vi "ISEG_HVSystem.ProcCases.vi"(0 "i ref in":refnum<vi>, 1 "selector":string, 2 "Data":T1, 3 "call cluster":T2={"Object"="", "Selector"="", "CallType"=enum."synchronous", "Async Object"="", "Async Selector"="", "Data Descriptor"="", "Data"=[], "Error #"=0, "Expire"=0}, 5 "error in (no error)":errorcluster) -> (14 "i ref out":refnum<vi>, 17 "answer cluster":T2={"Object"="", "Selector"="", "CallType"=enum."synchronous", "Async Object"="", "Async Selector"="", "Data Descriptor"="", "Data"=[], "Error #"=0, "Expire"=0}, 19 "error out":errorcluster)   [LabVIEW 2014, in "ISEG_HVSystem.lvlib"]
doc: "This method is called by a process from within the default case in the event loop. The methods of a class that are linked to events will be called from THIS method. Add your code here."
uses:
  ISEG_HVSystem.lvlib
  CSCore/CSSystem/CoreDefs/CoreDefs.call_type.ctl
  CSCore/BaseProcess/BaseProcess.descriptor string definition.ctl
  CSCore/CSSystem/CoreDefs/CoreDefs.rawDataType.ctl
  CSCore/CSSystem/CoreLib/CoreLib.byte array 2 string.vi
  CSCore/CSSystem/CoreLib/CoreLib.string 2 byte array.vi
  CSCore/CSSystem/CoreLib/CoreLib.byte array 2 short.vi
  CSCore/CSSystem/CoreLib/CoreLib.short 2 byte array.vi
  CSCore/CSSystem/CoreLib/CoreLib.byte array 2 double.vi
  CSCore/CSSystem/CoreLib/CoreLib.double 2 byte array.vi
  CSCore/CSApplicationBaseClasses/DeviceBase/DeviceBase.lvlib
  CSCore/CSSystem/CoreLib/CoreLib.lvlib
  CSCore/BaseProcess/BaseProcess.lvlib
  CSCore/CAEObj/CAEObj.lvlib
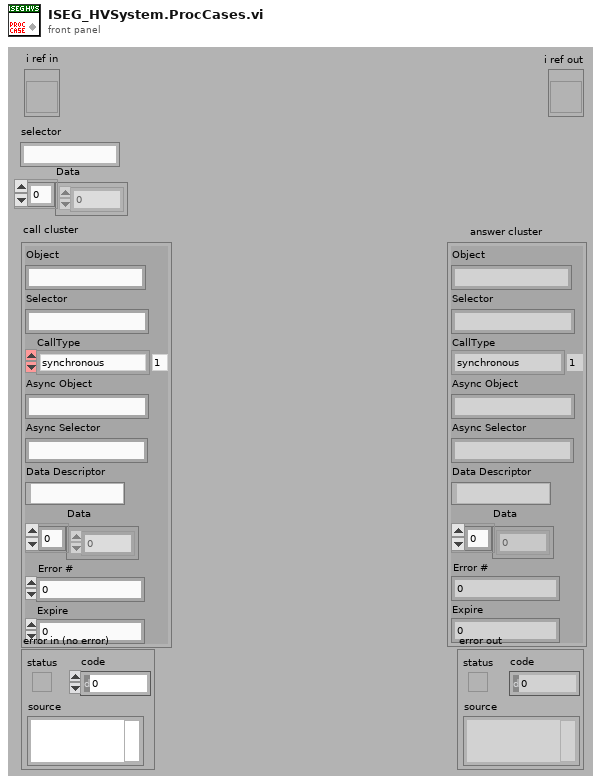
[diagram p1: front panel]
types:
  T1 = typedef "CoreDefs.rawDataType.ctl" = i8[]
  T2 = typedef "CoreDefs.call_type.ctl" = cluster{"Object":string, "Selector":string, "CallType":enum16{"simple", "synchronous", "asynchronous"}, "Async Object":string, "Async Selector":string, "Data Descriptor":T3, "Data":T1, "Error #":i32, "Expire":u32}
  T3 = typedef "BaseProcess.lvlib/BaseProcess.descriptor string definition.ctl" = string
  T4 = typedef "BaseProcess.lvlib/BaseProcess.i attribute.ctl" = cluster{"EventStatus":string, "EventError":i32, "PresetEvtWatchD":i32, "PresetPdcWatchD":i32, "EventTimeout":i32, "PeriodicInterval":i32, "Interface":string[], "Address":string[], "Special":string[], "PeriodicError":i32, "PeriodicStatus":string, "SuperProc":string, "Descriptors":T5[], "CaseRef":refnum<vi>, "PdcRef":refnum<vi>, "Thread Ref":refnum<vi>, "eventErrorID":i32, "eventStatusID":i32, "periodicErrorID":i32, "periodicStatusID":i32, "pdcCtrID":i32}
  T5 = typedef "BaseProcess.lvlib/BaseProcess.descriptor definition.ctl" = cluster{"selector":string, "descriptor":T3}
  T6 = typedef "ISEG_HVSystem.lvlib/ISEG_HVSystem.i attribute.ctl" = cluster{"System Name":string, "CAN_Status bus":cluster{"CAN":string, "DIM Status":T7}, "Client Active?":cluster{"Active":bool, "DIM Status":T7}, "Client Connected?":cluster{"Connected":bool, "DIM Status":T7}, "OPC Version":cluster{"OPC Version":string, "DIM Status":T7}, "Pr ID":cluster{"Pr ID":string, "DIM Status":T7}, " Modell":string, " Prefix":string, "Force":cluster{"Force":bool, "DIM Status":T7}, "Refresh":cluster{"Refresh":dbl, "DIM Status":T7}}
  T7 = typedef "ISEG_HVSystem.lvlib/ISEG_HVSystem.DIM Status.ctl" = cluster{"no link":bool, "quality":i32, "Time Stamp":timestamp}
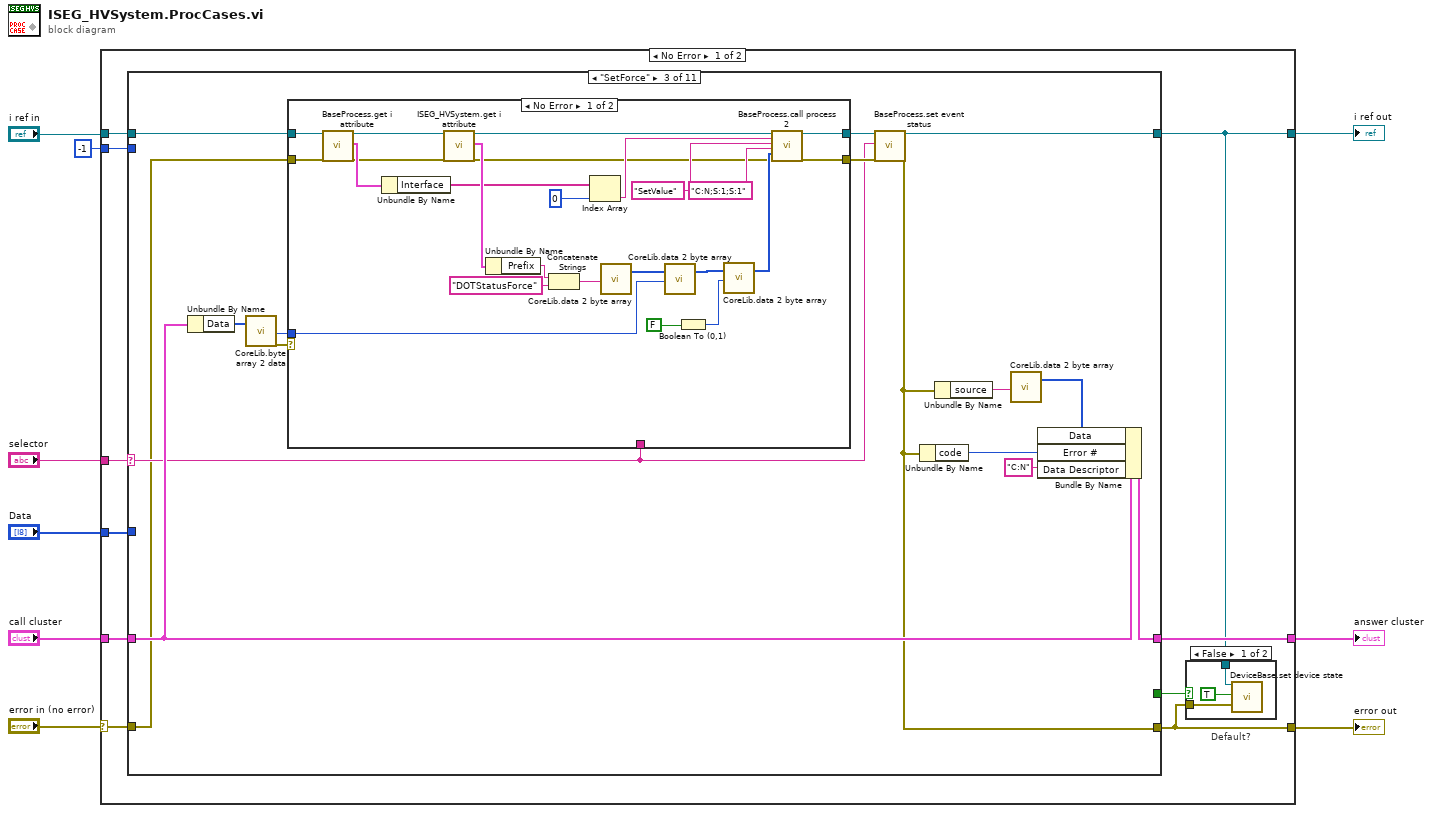
[diagram p0: block diagram]
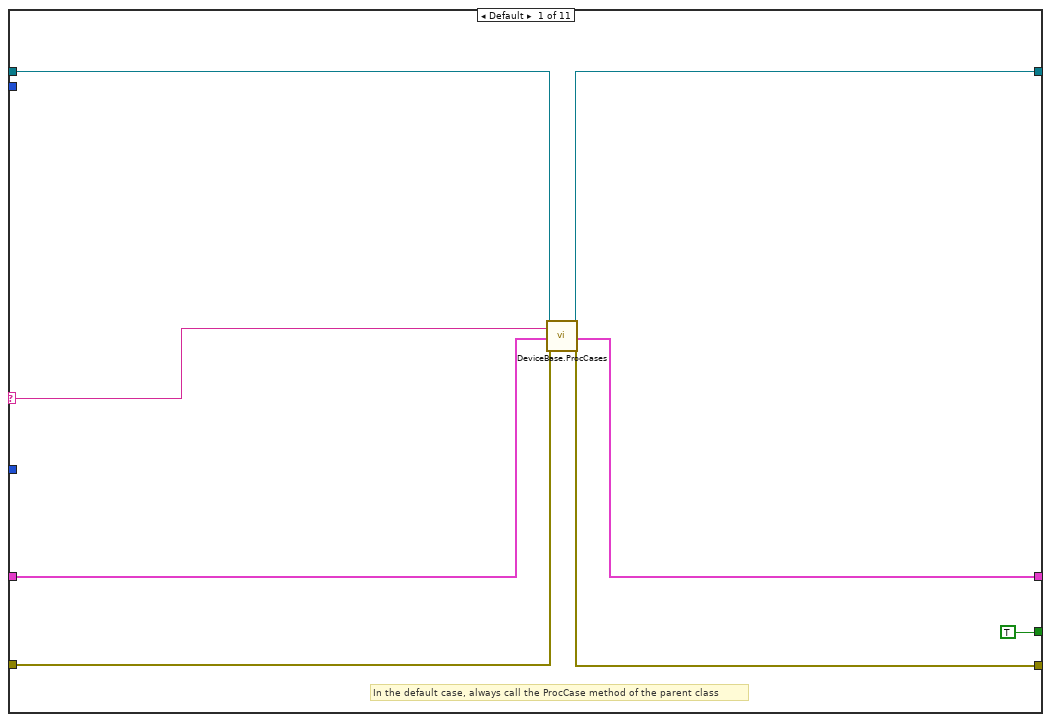
[diagram p3: hidden frame]
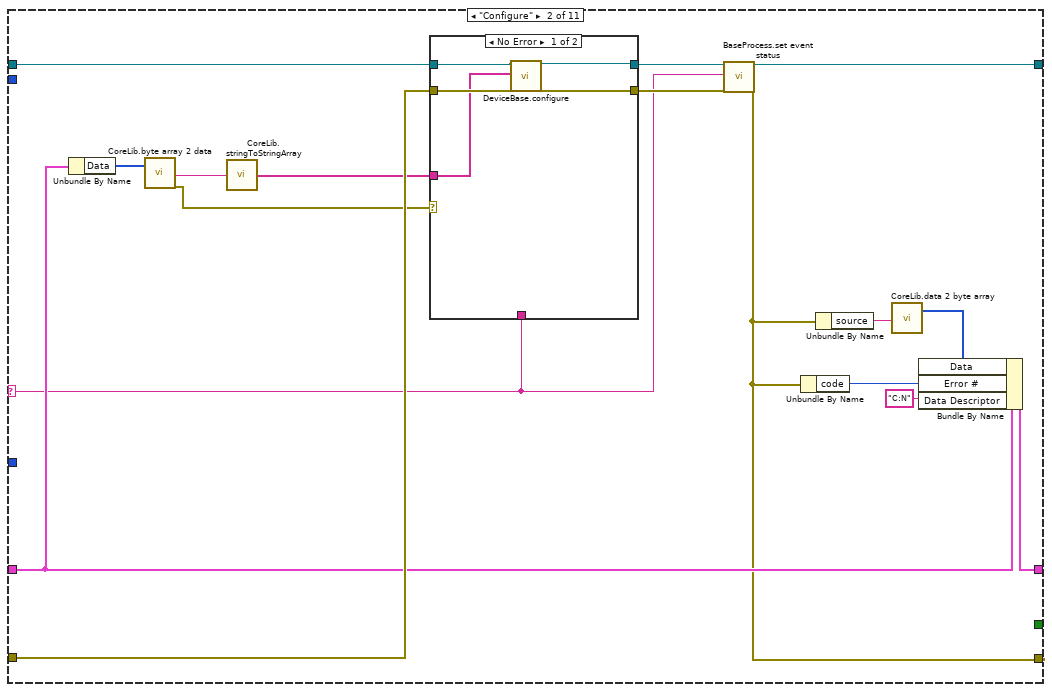
[diagram p4: hidden frame]
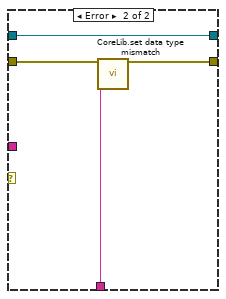
[diagram p5: hidden frame]
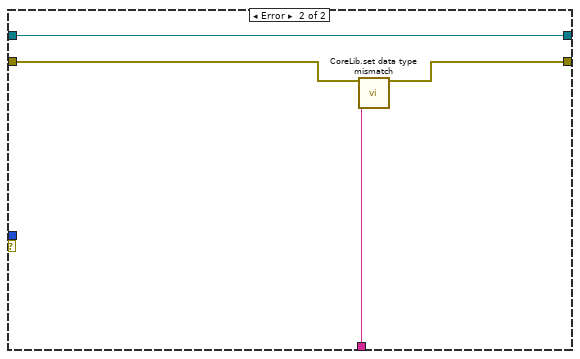
[diagram p6: hidden frame]
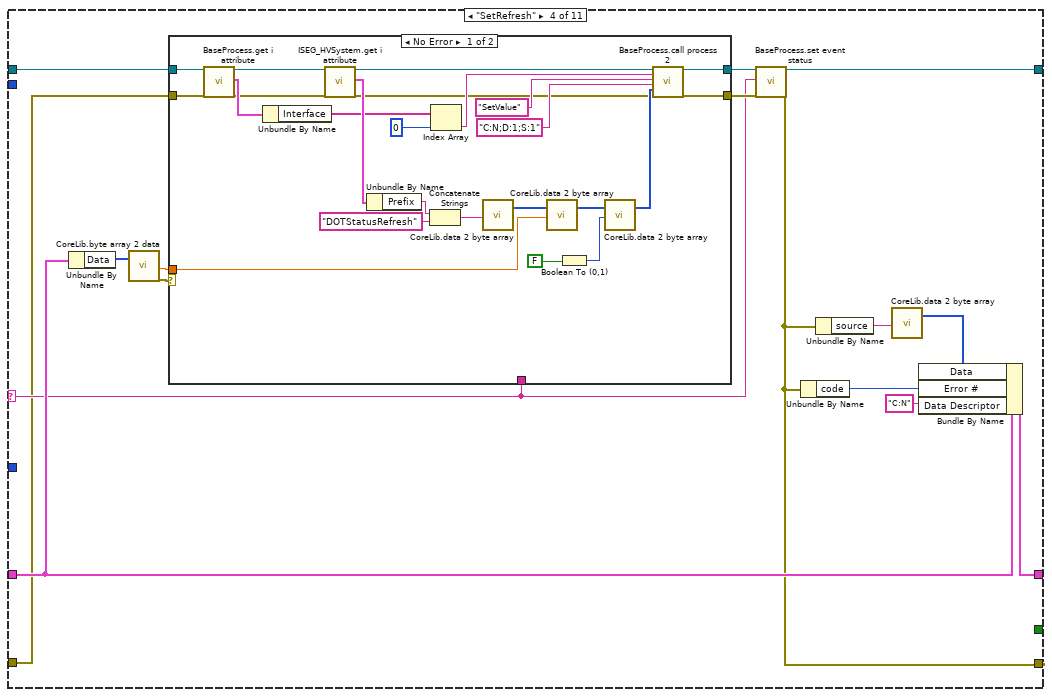
[diagram p7: hidden frame]
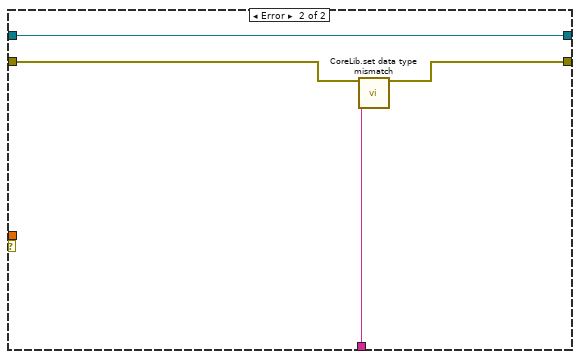
[diagram p8: hidden frame]
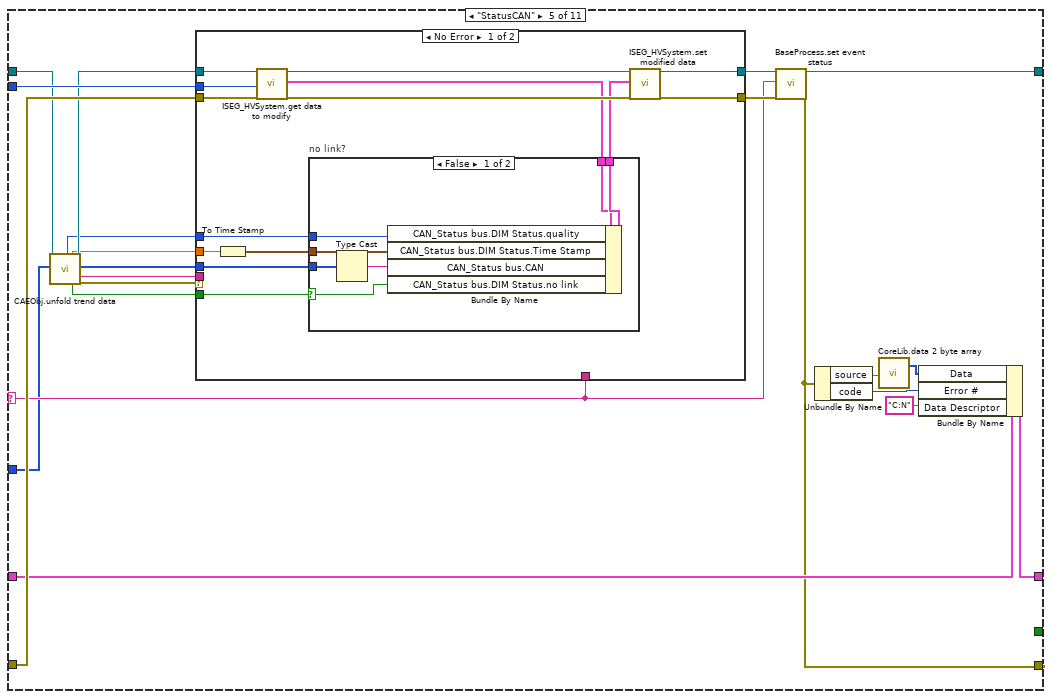
[diagram p9: hidden frame]
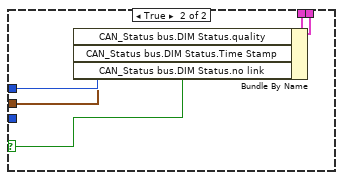
[diagram p10: hidden frame]
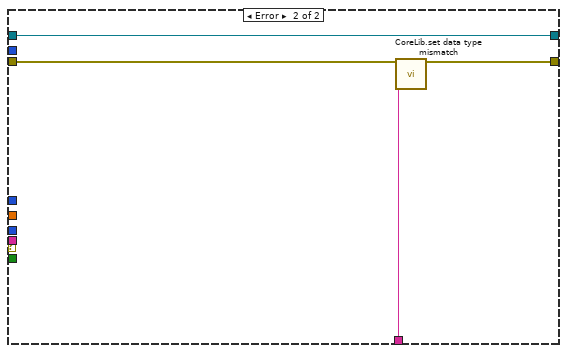
[diagram p11: hidden frame]
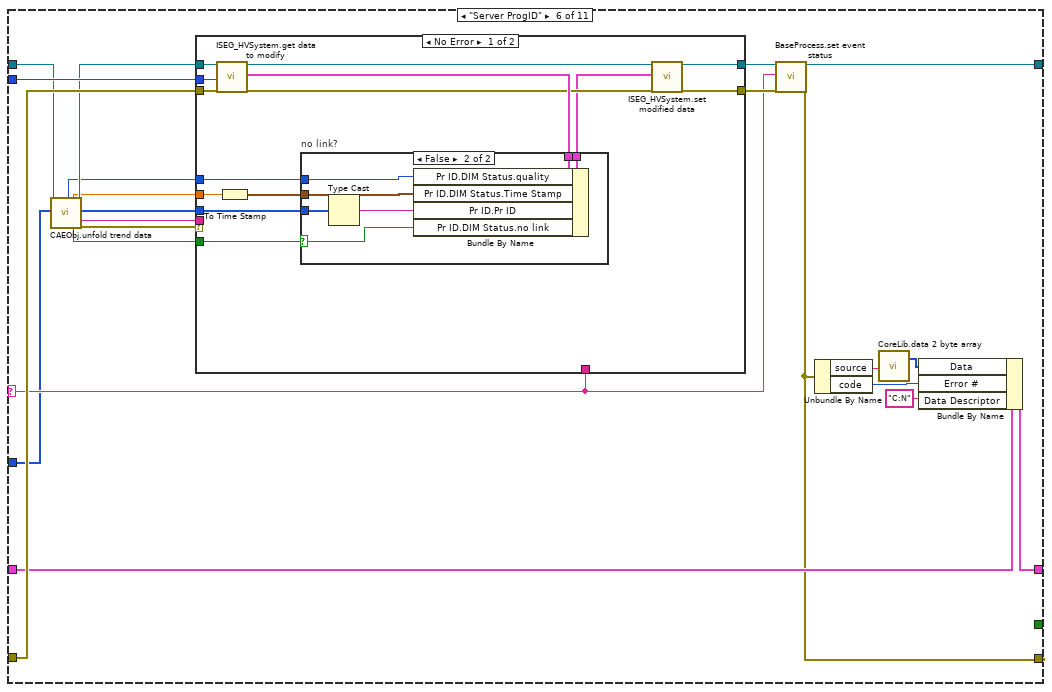
[diagram p12: hidden frame]
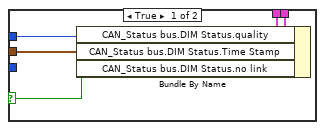
[diagram p13: hidden frame]
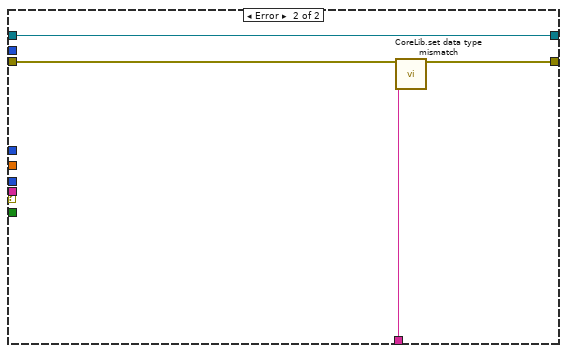
[diagram p14: hidden frame]
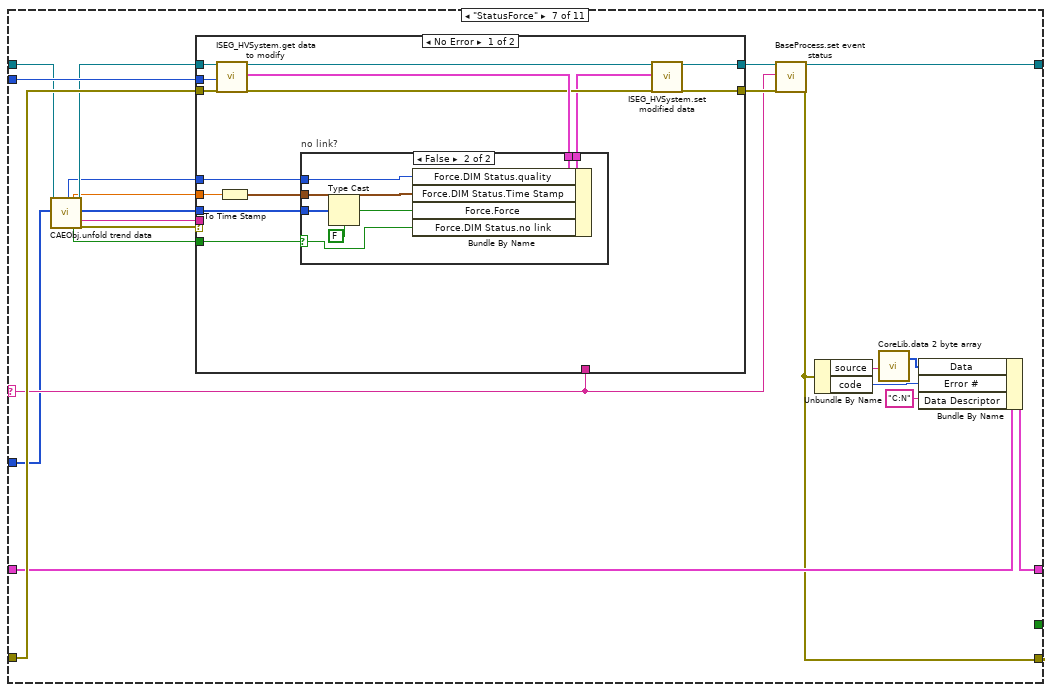
[diagram p15: hidden frame]
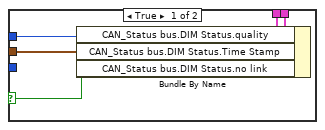
[diagram p16: hidden frame]
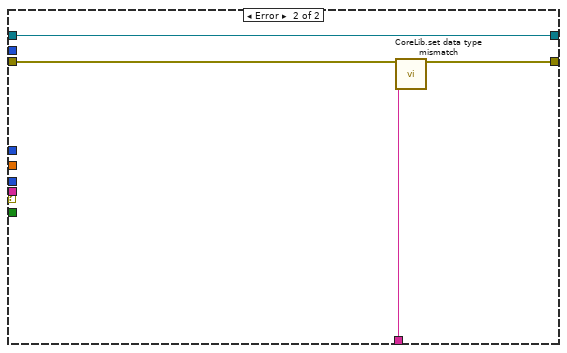
[diagram p17: hidden frame]
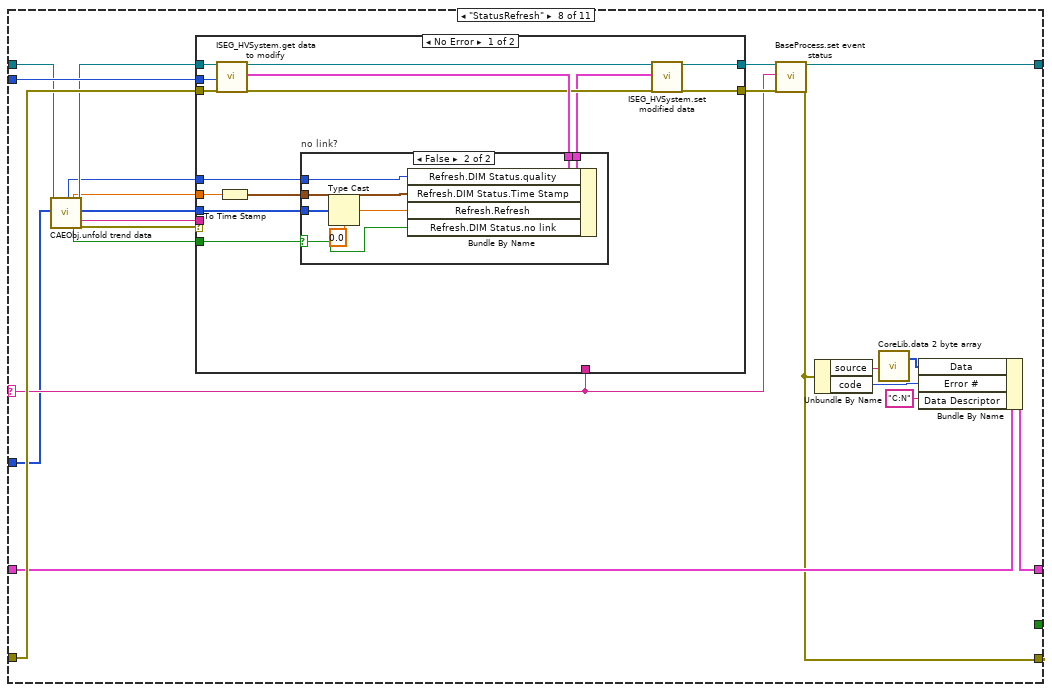
[diagram p18: hidden frame]
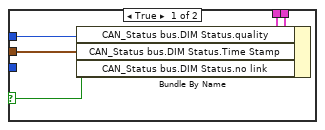
[diagram p19: hidden frame]
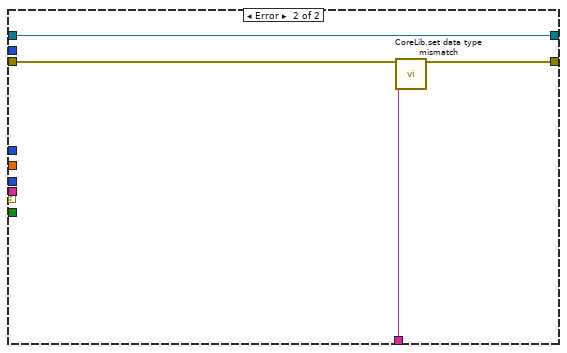
[diagram p20: hidden frame]
diagram:
  n1 = case shown="No Error" "error in (no error)" {
    selector: "error in (no error)" -> [w14 w512]
    tunnel: "selector" -> [w19 _]
    tunnel: [w18 w513] -> w3
    tunnel: "Data" -> [w17 _]
    tunnel: "call cluster" -> [w16 w513]
    tunnel: "i ref in" -> [w15 w514]
    tunnel: [w10 w514] -> w1
    tunnel: [w12 w512] -> w2
    tunnel: -1 ("ms timeout (10000)") -> [w13 _]
    frame No Error {
      n2 = case shown="\"SetForce\"" w19 {
        selector: w19 -> [w25 w38 w63 w107 w157 w209 w261 w314 w367 w419 w472]
        tunnel: w17 -> [_ _ _ _ w153 w205 w257 w310 w363 w415 w468]
        tunnel: w15 -> [w24 w47 w71 w115 w152 w204 w256 w309 w362 w414 w467]
        tunnel: [w30 w37 w62 w106 w156 w208 w260 w313 w366 w418 w471] -> w10
        tunnel: w16 -> [w26 w44 w69 w113 w163 w215 w267 w320 w373 w425 w478]
        tunnel: [w27 w43 w68 w112 w162 w214 w266 w319 w372 w424 w477] -> w18
        tunnel: w14 -> [w29 w46 w59 w103 w165 w217 w269 w322 w375 w427 w480]
        tunnel: [w28 w39 w64 w108 w158 w210 w262 w315 w368 w420 w473] -> w12
        tunnel: w13 -> [_ _ _ _ w154 w206 w258 w311 w364 w416 w469]
        tunnel: [TRUE _ _ _ _ _ _ _ _ _ _] -> w11
        frame Default {
          # "In the default case, always call the ProcCase method of the parent class"
          n3 = call "DeviceBase.ProcCases.vi"("i ref in"=w24, "selector"=w25, "call cluster"=w26, "error in (no error)"=w29) -> ("i ref out"=w30:refnum<vi>, "answer cluster"=w27:T2, "error out"=w28:errorcluster)  [unwired: 13 in]
        }
        frame "Configure" {
          n4 = Unbundle By Name(w44) -> ("Data"=w35:T1)
          n5 = call-poly "CoreLib.byte array 2 data.vi"("byteArray"=w35) -> ("string"=w32:string, "error out"=w33:errorcluster)  [unwired: 16 in, 1 out]
          n6 = call "CoreLib.stringToStringArray.vi"("String"=w32) -> ("Array"=w31:string[])
          n7 = case shown="No Error" w33 {
            tunnel: [w49 w55] -> w41
            tunnel: w47 -> [w50 w55]
            tunnel: w46 -> [w51 w54]
            tunnel: [w51 w53] -> w40
            tunnel: w38 -> [_ w52]
            tunnel: w31 -> [w48 _]
            frame No Error {
              n8 = call "DeviceBase.configure.vi"("i ref in"=w50, "configureData"=w48) -> ("i ref out"=w49:refnum<vi>)  [unwired: 15 in, 2 out]
            }
            frame Error {
              n9 = call "CoreLib.set data type mismatch.vi"("error in (no error)"=w54, "error source"=w52) -> ("error out"=w53:errorcluster)  [unwired: 17 in]
            }
          }
          n10 = call "BaseProcess.set event status.vi"("i ref in"=w41, "EventStatus"=w38, "error in (no error)"=w40) -> ("i ref out"=w37:refnum<vi>, "error out"=w39:errorcluster)  [unwired: 14 in, 1 out]
          n11 = Unbundle By Name(w39) -> ("code"=w45:i32)
          n12 = Unbundle By Name(w39) -> ("source"=w34:string)
          n13 = call-poly "CoreLib.data 2 byte array.vi"("string"=w34) -> ("byteArray out"=w42:T1)  [unwired: 18 in]
          n14 = Bundle By Name(cluster=w44, "Data"=w42, "Error #"=w45, "Data Descriptor"="C:N") -> (w43:T2)
        }
        frame "SetForce" {
          n15 = Unbundle By Name(w69) -> ("Data"=w58:T1)
          n16 = call-poly "CoreLib.byte array 2 data.vi"("byteArray"=w58) -> ("i16"=w57:i16, "error out"=w56:errorcluster)  [unwired: 16 in, 1 out]
          n17 = case shown="No Error" w56 {
            tunnel: [w78 w99] -> w66
            tunnel: w71 -> [w95 w99]
            tunnel: w59 -> [w94 w98]
            tunnel: [w79 w97] -> w65
            tunnel: w63 -> [_ w96]
            tunnel: w57 -> [w73 _]
            frame No Error {
              n18 = call "BaseProcess.get i attribute.vi"("i ref in"=w95, "error in (no error)"=w94) -> ("i ref out"=w92:refnum<vi>, "i attribute"=w93:T4, "error out"=w91:errorcluster)  [unwired: 15 in]
              n19 = Unbundle By Name(w93) -> ("Interface"=w84:string[])
              n20 = call "ISEG_HVSystem.get i attribute.vi"("i ref in"=w92, "error in (no error)"=w91) -> ("i ref out"=w77:refnum<vi>, "i attribute"=w90:T6, "error out"=w80:errorcluster)  [unwired: 15 in]
              n21 = Unbundle By Name(w90) -> ("Prefix"=w89:string)
              n22 = Concatenate Strings(w89, "DOTStatusForce" ("string")) -> (w87:string)
              n23 = Index Array(array=w84, index=0) -> (element=w85:string)
              n24 = call-poly "CoreLib.data 2 byte array.vi"("string"=w87) -> ("byteArray out"=w74:T1)  [unwired: 18 in]
              n25 = call-poly "CoreLib.data 2 byte array.vi"("byteArray"=w74, "i16"=w73) -> ("byteArray out"=w72:T1)  [unwired: 17 in]
              n26 = Boolean To (0,1)(Boolean=FALSE) -> (0, 1=w75:i16)
              n27 = call-poly "CoreLib.data 2 byte array.vi"("byteArray"=w72, "i16"=w75) -> ("byteArray out"=w81:T1)  [unwired: 17 in]
              n28 = call "BaseProcess.call process 2.vi"("i ref in"=w77, "Object"=w85, "Selector"="SetValue", "Data Descriptor"="C:N;S:1;S:1", "Data"=w81, "error in (no error)"=w80) -> ("i ref out"=w78:refnum<vi>, "error out"=w79:errorcluster)  [unwired: 12 in]
            }
            frame Error {
              n29 = call "CoreLib.set data type mismatch.vi"("error in (no error)"=w98, "error source"=w96) -> ("error out"=w97:errorcluster)  [unwired: 17 in]
            }
          }
          n30 = call "BaseProcess.set event status.vi"("i ref in"=w66, "EventStatus"=w63, "error in (no error)"=w65) -> ("i ref out"=w62:refnum<vi>, "error out"=w64:errorcluster)  [unwired: 14 in, 1 out]
          n31 = Unbundle By Name(w64) -> ("code"=w70:i32)
          n32 = Unbundle By Name(w64) -> ("source"=w60:string)
          n33 = call-poly "CoreLib.data 2 byte array.vi"("string"=w60) -> ("byteArray out"=w67:T1)  [unwired: 18 in]
          n34 = Bundle By Name(cluster=w69, "Data"=w67, "Error #"=w70, "Data Descriptor"="C:N") -> (w68:T2)
        }
        frame "SetRefresh" {
          n35 = Unbundle By Name(w113) -> ("Data"=w100:T1)
          n36 = call-poly "CoreLib.byte array 2 data.vi"("byteArray"=w100) -> ("d64"=w102:dbl, "error out"=w101:errorcluster)  [unwired: 16 in, 1 out]
          n37 = case shown="No Error" w101 {
            tunnel: [w122 w143] -> w110
            tunnel: w115 -> [w139 w143]
            tunnel: w103 -> [w138 w142]
            tunnel: [w123 w141] -> w109
            tunnel: w107 -> [_ w140]
            tunnel: w102 -> [w116 _]
            frame No Error {
              n38 = call "BaseProcess.get i attribute.vi"("i ref in"=w139, "error in (no error)"=w138) -> ("i ref out"=w136:refnum<vi>, "i attribute"=w137:T4, "error out"=w135:errorcluster)  [unwired: 15 in]
              n39 = Unbundle By Name(w137) -> ("Interface"=w128:string[])
              n40 = call "ISEG_HVSystem.get i attribute.vi"("i ref in"=w136, "error in (no error)"=w135) -> ("i ref out"=w121:refnum<vi>, "i attribute"=w134:T6, "error out"=w124:errorcluster)  [unwired: 15 in]
              n41 = Unbundle By Name(w134) -> ("Prefix"=w133:string)
              n42 = Concatenate Strings(w133, "DOTStatusRefresh" ("string")) -> (w131:string)
              n43 = Index Array(array=w128, index=0) -> (element=w129:string)
              n44 = call-poly "CoreLib.data 2 byte array.vi"("string"=w131) -> ("byteArray out"=w118:T1)  [unwired: 18 in]
              n45 = call-poly "CoreLib.data 2 byte array.vi"("byteArray"=w118, "f64"=w116) -> ("byteArray out"=w117:T1)  [unwired: 17 in]
              n46 = Boolean To (0,1)(Boolean=FALSE) -> (0, 1=w119:i16)
              n47 = call-poly "CoreLib.data 2 byte array.vi"("byteArray"=w117, "i16"=w119) -> ("byteArray out"=w125:T1)  [unwired: 17 in]
              n48 = call "BaseProcess.call process 2.vi"("i ref in"=w121, "Object"=w129, "Selector"="SetValue", "Data Descriptor"="C:N;D:1;S:1", "Data"=w125, "error in (no error)"=w124) -> ("i ref out"=w122:refnum<vi>, "error out"=w123:errorcluster)  [unwired: 12 in]
            }
            frame Error {
              n49 = call "CoreLib.set data type mismatch.vi"("error in (no error)"=w142, "error source"=w140) -> ("error out"=w141:errorcluster)  [unwired: 17 in]
            }
          }
          n50 = call "BaseProcess.set event status.vi"("i ref in"=w110, "EventStatus"=w107, "error in (no error)"=w109) -> ("i ref out"=w106:refnum<vi>, "error out"=w108:errorcluster)  [unwired: 14 in, 1 out]
          n51 = Unbundle By Name(w108) -> ("code"=w114:i32)
          n52 = Unbundle By Name(w108) -> ("source"=w104:string)
          n53 = call-poly "CoreLib.data 2 byte array.vi"("string"=w104) -> ("byteArray out"=w111:T1)  [unwired: 18 in]
          n54 = Bundle By Name(cluster=w113, "Data"=w111, "Error #"=w114, "Data Descriptor"="C:N") -> (w112:T2)
        }
        frame "StatusCAN" {
          n55 = call "CAEObj.unfold trend data.vi"("i ref in"=w152, "raw trend data"=w153) -> ("quality"=w146:i32, "timeStamp"=w145:dbl, "no link"=w147:bool, "i ref out"=w151:refnum<vi>, "data"=w150:i8[], "typeDescriptor"=w148:string, "error out"=w144:errorcluster)  [unwired: 9 in, 2 out]
          n56 = case shown="No Error" w144 {
            tunnel: [w171 w195] -> w160
            tunnel: w151 -> [w179 w195]
            tunnel: w165 -> [w178 w194]
            tunnel: [w170 w193] -> w159
            tunnel: w157 -> [_ w192]
            tunnel: w154 -> [w177 _]
            tunnel: w150 -> [w173 _]
            tunnel: w148 -> [_ _]
            tunnel: w147 -> [w166 _]
            tunnel: w146 -> [w169 _]
            tunnel: w145 -> [w168 _]
            frame No Error {
              n57 = To Time Stamp(1:w168) -> (0:w167:timestamp)
              n58 = call "ISEG_HVSystem.get data to modify.vi"("i ref in"=w179, "ms timeout (10000)"=w177, "error in (no error)"=w178) -> ("i ref out"=w176:refnum<vi>, "i attribute"=w172:T6, "error out"=w175:errorcluster)  [unwired: 13 in, 1 out]
              n59 = case "no link?" shown="False" w166 {
                selector: w166 -> [w180 w187]
                tunnel: [w186 w191] -> w174
                tunnel: w173 -> [w185 _]
                tunnel: w172 -> [w183 w190]
                tunnel: w169 -> [w182 w189]
                tunnel: w167 -> [w181 w188]
                frame False {
                  n60 = Type Cast(x=w185) -> (*(type *) &x=w184:string)  [unwired: 1 in]
                  n61 = Bundle By Name(cluster=w183, "CAN_Status bus.DIM Status.quality"=w182, "CAN_Status bus.DIM Status.Time Stamp"=w181, "CAN_Status bus.CAN"=w184, "CAN_Status bus.DIM Status.no link"=w180) -> (w186:T6)
                }
                frame True {
                  n62 = Bundle By Name(cluster=w190, "CAN_Status bus.DIM Status.quality"=w189, "CAN_Status bus.DIM Status.Time Stamp"=w188, "CAN_Status bus.DIM Status.no link"=w187) -> (w191:T6)
                }
              }
              n63 = call "ISEG_HVSystem.set modified data.vi"("i ref in"=w176, "i attribute"=w174, "error in (no error)"=w175) -> ("i ref out"=w171:refnum<vi>, "error out"=w170:errorcluster)  [unwired: 15 in]
            }
            frame Error {
              n64 = call "CoreLib.set data type mismatch.vi"("error in (no error)"=w194, "error source"=w192) -> ("error out"=w193:errorcluster)  [unwired: 17 in]
            }
          }
          n65 = call "BaseProcess.set event status.vi"("i ref in"=w160, "EventStatus"=w157, "error in (no error)"=w159) -> ("i ref out"=w156:refnum<vi>, "error out"=w158:errorcluster)  [unwired: 14 in, 1 out]
          n66 = Unbundle By Name(w158) -> ("source"=w149:string, "code"=w164:i32)
          n67 = call-poly "CoreLib.data 2 byte array.vi"("string"=w149) -> ("byteArray out"=w161:T1)  [unwired: 18 in]
          n68 = Bundle By Name(cluster=w163, "Data"=w161, "Error #"=w164, "Data Descriptor"="C:N") -> (w162:T2)
        }
        frame "Server ProgID" {
          n69 = call "CAEObj.unfold trend data.vi"("i ref in"=w204, "raw trend data"=w205) -> ("quality"=w197:i32, "timeStamp"=w196:dbl, "no link"=w198:bool, "i ref out"=w203:refnum<vi>, "data"=w202:i8[], "typeDescriptor"=w200:string, "error out"=w199:errorcluster)  [unwired: 9 in, 2 out]
          n70 = case shown="No Error" w199 {
            tunnel: [w224 w247] -> w212
            tunnel: w203 -> [w231 w247]
            tunnel: w217 -> [w230 w246]
            tunnel: [w225 w245] -> w211
            tunnel: w209 -> [_ w244]
            tunnel: w206 -> [w229 _]
            tunnel: w202 -> [w222 _]
            tunnel: w200 -> [_ _]
            tunnel: w198 -> [w218 _]
            tunnel: w197 -> [w221 _]
            tunnel: w196 -> [w220 _]
            frame No Error {
              n71 = call "ISEG_HVSystem.get data to modify.vi"("i ref in"=w231, "ms timeout (10000)"=w229, "error in (no error)"=w230) -> ("i ref out"=w227:refnum<vi>, "i attribute"=w228:T6, "error out"=w226:errorcluster)  [unwired: 13 in, 1 out]
              n72 = To Time Stamp(1:w220) -> (0:w219:timestamp)
              n73 = case "no link?" shown="False" w218 {
                selector: w218 -> [w232 w237]
                tunnel: w228 -> [w236 w243]
                tunnel: [w235 w242] -> w223
                tunnel: w222 -> [_ w241]
                tunnel: w221 -> [w234 w239]
                tunnel: w219 -> [w233 w238]
                frame True {
                  n74 = Bundle By Name(cluster=w236, "CAN_Status bus.DIM Status.quality"=w234, "CAN_Status bus.DIM Status.Time Stamp"=w233, "CAN_Status bus.DIM Status.no link"=w232) -> (w235:T6)
                }
                frame False {
                  n75 = Type Cast(x=w241) -> (*(type *) &x=w240:string)  [unwired: 1 in]
                  n76 = Bundle By Name(cluster=w243, "Pr ID.DIM Status.quality"=w239, "Pr ID.DIM Status.Time Stamp"=w238, "Pr ID.Pr ID"=w240, "Pr ID.DIM Status.no link"=w237) -> (w242:T6)
                }
              }
              n77 = call "ISEG_HVSystem.set modified data.vi"("i ref in"=w227, "i attribute"=w223, "error in (no error)"=w226) -> ("i ref out"=w224:refnum<vi>, "error out"=w225:errorcluster)  [unwired: 15 in]
            }
            frame Error {
              n78 = call "CoreLib.set data type mismatch.vi"("error in (no error)"=w246, "error source"=w244) -> ("error out"=w245:errorcluster)  [unwired: 17 in]
            }
          }
          n79 = call "BaseProcess.set event status.vi"("i ref in"=w212, "EventStatus"=w209, "error in (no error)"=w211) -> ("i ref out"=w208:refnum<vi>, "error out"=w210:errorcluster)  [unwired: 14 in, 1 out]
          n80 = Unbundle By Name(w210) -> ("source"=w201:string, "code"=w216:i32)
          n81 = call-poly "CoreLib.data 2 byte array.vi"("string"=w201) -> ("byteArray out"=w213:T1)  [unwired: 18 in]
          n82 = Bundle By Name(cluster=w215, "Data"=w213, "Error #"=w216, "Data Descriptor"="C:N") -> (w214:T2)
        }
        frame "StatusForce" {
          n83 = call "CAEObj.unfold trend data.vi"("i ref in"=w256, "raw trend data"=w257) -> ("quality"=w249:i32, "timeStamp"=w248:dbl, "no link"=w250:bool, "i ref out"=w255:refnum<vi>, "data"=w254:i8[], "typeDescriptor"=w252:string, "error out"=w251:errorcluster)  [unwired: 9 in, 2 out]
          n84 = case shown="No Error" w251 {
            tunnel: [w276 w300] -> w264
            tunnel: w255 -> [w283 w300]
            tunnel: w269 -> [w282 w299]
            tunnel: [w277 w298] -> w263
            tunnel: w261 -> [_ w297]
            tunnel: w258 -> [w281 _]
            tunnel: w254 -> [w274 _]
            tunnel: w252 -> [_ _]
            tunnel: w250 -> [w270 _]
            tunnel: w249 -> [w273 _]
            tunnel: w248 -> [w272 _]
            frame No Error {
              n85 = call "ISEG_HVSystem.get data to modify.vi"("i ref in"=w283, "ms timeout (10000)"=w281, "error in (no error)"=w282) -> ("i ref out"=w279:refnum<vi>, "i attribute"=w280:T6, "error out"=w278:errorcluster)  [unwired: 13 in, 1 out]
              n86 = To Time Stamp(1:w272) -> (0:w271:timestamp)
              n87 = case "no link?" shown="False" w270 {
                selector: w270 -> [w284 w291]
                tunnel: w280 -> [w288 w296]
                tunnel: [w287 w295] -> w275
                tunnel: w274 -> [_ w294]
                tunnel: w273 -> [w286 w293]
                tunnel: w271 -> [w285 w292]
                frame True {
                  n88 = Bundle By Name(cluster=w288, "CAN_Status bus.DIM Status.quality"=w286, "CAN_Status bus.DIM Status.Time Stamp"=w285, "CAN_Status bus.DIM Status.no link"=w284) -> (w287:T6)
                }
                frame False {
                  n89 = Type Cast(type=FALSE, x=w294) -> (*(type *) &x=w289:bool)
                  n90 = Bundle By Name(cluster=w296, "Force.DIM Status.quality"=w293, "Force.DIM Status.Time Stamp"=w292, "Force.Force"=w289, "Force.DIM Status.no link"=w291) -> (w295:T6)
                }
              }
              n91 = call "ISEG_HVSystem.set modified data.vi"("i ref in"=w279, "i attribute"=w275, "error in (no error)"=w278) -> ("i ref out"=w276:refnum<vi>, "error out"=w277:errorcluster)  [unwired: 15 in]
            }
            frame Error {
              n92 = call "CoreLib.set data type mismatch.vi"("error in (no error)"=w299, "error source"=w297) -> ("error out"=w298:errorcluster)  [unwired: 17 in]
            }
          }
          n93 = call "BaseProcess.set event status.vi"("i ref in"=w264, "EventStatus"=w261, "error in (no error)"=w263) -> ("i ref out"=w260:refnum<vi>, "error out"=w262:errorcluster)  [unwired: 14 in, 1 out]
          n94 = Unbundle By Name(w262) -> ("source"=w253:string, "code"=w268:i32)
          n95 = call-poly "CoreLib.data 2 byte array.vi"("string"=w253) -> ("byteArray out"=w265:T1)  [unwired: 18 in]
          n96 = Bundle By Name(cluster=w267, "Data"=w265, "Error #"=w268, "Data Descriptor"="C:N") -> (w266:T2)
        }
        frame "StatusRefresh" {
          n97 = call "CAEObj.unfold trend data.vi"("i ref in"=w309, "raw trend data"=w310) -> ("quality"=w302:i32, "timeStamp"=w301:dbl, "no link"=w303:bool, "i ref out"=w308:refnum<vi>, "data"=w307:i8[], "typeDescriptor"=w305:string, "error out"=w304:errorcluster)  [unwired: 9 in, 2 out]
          n98 = case shown="No Error" w304 {
            tunnel: [w329 w353] -> w317
            tunnel: w308 -> [w336 w353]
            tunnel: w322 -> [w335 w352]
            tunnel: [w330 w351] -> w316
            tunnel: w314 -> [_ w350]
            tunnel: w311 -> [w334 _]
            tunnel: w307 -> [w327 _]
            tunnel: w305 -> [_ _]
            tunnel: w303 -> [w323 _]
            tunnel: w302 -> [w326 _]
            tunnel: w301 -> [w325 _]
            frame No Error {
              n99 = call "ISEG_HVSystem.get data to modify.vi"("i ref in"=w336, "ms timeout (10000)"=w334, "error in (no error)"=w335) -> ("i ref out"=w332:refnum<vi>, "i attribute"=w333:T6, "error out"=w331:errorcluster)  [unwired: 13 in, 1 out]
              n100 = To Time Stamp(1:w325) -> (0:w324:timestamp)
              n101 = case "no link?" shown="False" w323 {
                selector: w323 -> [w337 w344]
                tunnel: w333 -> [w341 w349]
                tunnel: [w340 w348] -> w328
                tunnel: w327 -> [_ w347]
                tunnel: w326 -> [w339 w346]
                tunnel: w324 -> [w338 w345]
                frame True {
                  n102 = Bundle By Name(cluster=w341, "CAN_Status bus.DIM Status.quality"=w339, "CAN_Status bus.DIM Status.Time Stamp"=w338, "CAN_Status bus.DIM Status.no link"=w337) -> (w340:T6)
                }
                frame False {
                  n103 = Type Cast(type=0.0, x=w347) -> (*(type *) &x=w342:dbl)
                  n104 = Bundle By Name(cluster=w349, "Refresh.DIM Status.quality"=w346, "Refresh.DIM Status.Time Stamp"=w345, "Refresh.Refresh"=w342, "Refresh.DIM Status.no link"=w344) -> (w348:T6)
                }
              }
              n105 = call "ISEG_HVSystem.set modified data.vi"("i ref in"=w332, "i attribute"=w328, "error in (no error)"=w331) -> ("i ref out"=w329:refnum<vi>, "error out"=w330:errorcluster)  [unwired: 15 in]
            }
            frame Error {
              n106 = call "CoreLib.set data type mismatch.vi"("error in (no error)"=w352, "error source"=w350) -> ("error out"=w351:errorcluster)  [unwired: 17 in]
            }
          }
          n107 = call "BaseProcess.set event status.vi"("i ref in"=w317, "EventStatus"=w314, "error in (no error)"=w316) -> ("i ref out"=w313:refnum<vi>, "error out"=w315:errorcluster)  [unwired: 14 in, 1 out]
          n108 = Unbundle By Name(w315) -> ("source"=w306:string, "code"=w321:i32)
          n109 = call-poly "CoreLib.data 2 byte array.vi"("string"=w306) -> ("byteArray out"=w318:T1)  [unwired: 18 in]
          n110 = Bundle By Name(cluster=w320, "Data"=w318, "Error #"=w321, "Data Descriptor"="C:N") -> (w319:T2)
        }
        frame "OPC Interface Version" {
          n111 = call "CAEObj.unfold trend data.vi"("i ref in"=w362, "raw trend data"=w363) -> ("quality"=w354:i32, "timeStamp"=w355:dbl, "no link"=w356:bool, "i ref out"=w361:refnum<vi>, "data"=w360:i8[], "typeDescriptor"=w358:string, "error out"=w357:errorcluster)  [unwired: 9 in, 2 out]
          n112 = case shown="No Error" w357 {
            tunnel: [w382 w405] -> w370
            tunnel: w361 -> [w389 w405]
            tunnel: w375 -> [w388 w404]
            tunnel: [w383 w403] -> w369
            tunnel: w367 -> [_ w402]
            tunnel: w364 -> [w387 _]
            tunnel: w360 -> [w380 _]
            tunnel: w358 -> [_ _]
            tunnel: w356 -> [w376 _]
            tunnel: w355 -> [w379 _]
            tunnel: w354 -> [w377 _]
            frame No Error {
              n113 = call "ISEG_HVSystem.get data to modify.vi"("i ref in"=w389, "ms timeout (10000)"=w387, "error in (no error)"=w388) -> ("i ref out"=w385:refnum<vi>, "i attribute"=w386:T6, "error out"=w384:errorcluster)  [unwired: 13 in, 1 out]
              n114 = To Time Stamp(1:w379) -> (0:w378:timestamp)
              n115 = case "no link?" shown="False" w376 {
                selector: w376 -> [w390 w395]
                tunnel: w386 -> [w394 w401]
                tunnel: [w393 w400] -> w381
                tunnel: w380 -> [_ w399]
                tunnel: w378 -> [w392 w397]
                tunnel: w377 -> [w391 w396]
                frame True {
                  n116 = Bundle By Name(cluster=w394, "CAN_Status bus.DIM Status.quality"=w391, "CAN_Status bus.DIM Status.Time Stamp"=w392, "CAN_Status bus.DIM Status.no link"=w390) -> (w393:T6)
                }
                frame False {
                  n117 = Type Cast(x=w399) -> (*(type *) &x=w398:string)  [unwired: 1 in]
                  n118 = Bundle By Name(cluster=w401, "OPC Version.DIM Status.quality"=w396, "OPC Version.DIM Status.Time Stamp"=w397, "OPC Version.OPC Version"=w398, "OPC Version.DIM Status.no link"=w395) -> (w400:T6)
                }
              }
              n119 = call "ISEG_HVSystem.set modified data.vi"("i ref in"=w385, "i attribute"=w381, "error in (no error)"=w384) -> ("i ref out"=w382:refnum<vi>, "error out"=w383:errorcluster)  [unwired: 15 in]
            }
            frame Error {
              n120 = call "CoreLib.set data type mismatch.vi"("error in (no error)"=w404, "error source"=w402) -> ("error out"=w403:errorcluster)  [unwired: 17 in]
            }
          }
          n121 = call "BaseProcess.set event status.vi"("i ref in"=w370, "EventStatus"=w367, "error in (no error)"=w369) -> ("i ref out"=w366:refnum<vi>, "error out"=w368:errorcluster)  [unwired: 14 in, 1 out]
          n122 = Unbundle By Name(w368) -> ("source"=w359:string, "code"=w374:i32)
          n123 = call-poly "CoreLib.data 2 byte array.vi"("string"=w359) -> ("byteArray out"=w371:T1)  [unwired: 18 in]
          n124 = Bundle By Name(cluster=w373, "Data"=w371, "Error #"=w374, "Data Descriptor"="C:N") -> (w372:T2)
        }
        frame "Active" {
          n125 = call "CAEObj.unfold trend data.vi"("i ref in"=w414, "raw trend data"=w415) -> ("quality"=w409:i32, "timeStamp"=w408:dbl, "no link"=w406:bool, "i ref out"=w413:refnum<vi>, "data"=w412:i8[], "typeDescriptor"=w410:string, "error out"=w407:errorcluster)  [unwired: 9 in, 2 out]
          n126 = case shown="No Error" w407 {
            tunnel: [w434 w458] -> w422
            tunnel: w413 -> [w441 w458]
            tunnel: w427 -> [w440 w457]
            tunnel: [w435 w456] -> w421
            tunnel: w419 -> [_ w455]
            tunnel: w416 -> [w439 _]
            tunnel: w412 -> [w432 _]
            tunnel: w410 -> [_ _]
            tunnel: w409 -> [w431 _]
            tunnel: w408 -> [w429 _]
            tunnel: w406 -> [w428 _]
            frame No Error {
              n127 = To Time Stamp(1:w429) -> (0:w430:timestamp)
              n128 = call "ISEG_HVSystem.get data to modify.vi"("i ref in"=w441, "ms timeout (10000)"=w439, "error in (no error)"=w440) -> ("i ref out"=w437:refnum<vi>, "i attribute"=w438:T6, "error out"=w436:errorcluster)  [unwired: 13 in, 1 out]
              n129 = case "no link?" shown="False" w428 {
                selector: w428 -> [w442 w449]
                tunnel: w438 -> [w446 w454]
                tunnel: [w445 w453] -> w433
                tunnel: w432 -> [_ w452]
                tunnel: w431 -> [w444 w451]
                tunnel: w430 -> [w443 w450]
                frame True {
                  n130 = Bundle By Name(cluster=w446, "CAN_Status bus.DIM Status.quality"=w444, "CAN_Status bus.DIM Status.Time Stamp"=w443, "CAN_Status bus.DIM Status.no link"=w442) -> (w445:T6)
                }
                frame False {
                  n131 = Type Cast(type=FALSE, x=w452) -> (*(type *) &x=w447:bool)
                  n132 = Bundle By Name(cluster=w454, "Client Active?.DIM Status.quality"=w451, "Client Active?.DIM Status.Time Stamp"=w450, "Client Active?.Active"=w447, "Client Active?.DIM Status.no link"=w449) -> (w453:T6)
                }
              }
              n133 = call "ISEG_HVSystem.set modified data.vi"("i ref in"=w437, "i attribute"=w433, "error in (no error)"=w436) -> ("i ref out"=w434:refnum<vi>, "error out"=w435:errorcluster)  [unwired: 15 in]
            }
            frame Error {
              n134 = call "CoreLib.set data type mismatch.vi"("error in (no error)"=w457, "error source"=w455) -> ("error out"=w456:errorcluster)  [unwired: 17 in]
            }
          }
          n135 = call "BaseProcess.set event status.vi"("i ref in"=w422, "EventStatus"=w419, "error in (no error)"=w421) -> ("i ref out"=w418:refnum<vi>, "error out"=w420:errorcluster)  [unwired: 14 in, 1 out]
          n136 = Unbundle By Name(w420) -> ("source"=w411:string, "code"=w426:i32)
          n137 = call-poly "CoreLib.data 2 byte array.vi"("string"=w411) -> ("byteArray out"=w423:T1)  [unwired: 18 in]
          n138 = Bundle By Name(cluster=w425, "Data"=w423, "Error #"=w426, "Data Descriptor"="C:N") -> (w424:T2)
        }
        frame "Connected" {
          n139 = call "CAEObj.unfold trend data.vi"("i ref in"=w467, "raw trend data"=w468) -> ("quality"=w462:i32, "timeStamp"=w461:dbl, "no link"=w459:bool, "i ref out"=w466:refnum<vi>, "data"=w465:i8[], "typeDescriptor"=w463:string, "error out"=w460:errorcluster)  [unwired: 9 in, 2 out]
          n140 = case shown="No Error" w460 {
            tunnel: [w487 w511] -> w475
            tunnel: w466 -> [w494 w511]
            tunnel: w480 -> [w493 w510]
            tunnel: [w488 w509] -> w474
            tunnel: w472 -> [_ w508]
            tunnel: w469 -> [w492 _]
            tunnel: w465 -> [w485 _]
            tunnel: w463 -> [_ _]
            tunnel: w462 -> [w484 _]
            tunnel: w461 -> [w482 _]
            tunnel: w459 -> [w481 _]
            frame No Error {
              n141 = To Time Stamp(1:w482) -> (0:w483:timestamp)
              n142 = call "ISEG_HVSystem.get data to modify.vi"("i ref in"=w494, "ms timeout (10000)"=w492, "error in (no error)"=w493) -> ("i ref out"=w490:refnum<vi>, "i attribute"=w491:T6, "error out"=w489:errorcluster)  [unwired: 13 in, 1 out]
              n143 = case "no link?" shown="False" w481 {
                selector: w481 -> [w495 w502]
                tunnel: w491 -> [w499 w507]
                tunnel: [w498 w506] -> w486
                tunnel: w485 -> [_ w505]
                tunnel: w484 -> [w497 w504]
                tunnel: w483 -> [w496 w503]
                frame True {
                  n144 = Bundle By Name(cluster=w499, "CAN_Status bus.DIM Status.quality"=w497, "CAN_Status bus.DIM Status.Time Stamp"=w496, "CAN_Status bus.DIM Status.no link"=w495) -> (w498:T6)
                }
                frame False {
                  n145 = Type Cast(type=FALSE, x=w505) -> (*(type *) &x=w500:bool)
                  n146 = Bundle By Name(cluster=w507, "Client Connected?.DIM Status.quality"=w504, "Client Connected?.DIM Status.Time Stamp"=w503, "Client Connected?.Connected"=w500, "Client Connected?.DIM Status.no link"=w502) -> (w506:T6)
                }
              }
              n147 = call "ISEG_HVSystem.set modified data.vi"("i ref in"=w490, "i attribute"=w486, "error in (no error)"=w489) -> ("i ref out"=w487:refnum<vi>, "error out"=w488:errorcluster)  [unwired: 15 in]
            }
            frame Error {
              n148 = call "CoreLib.set data type mismatch.vi"("error in (no error)"=w510, "error source"=w508) -> ("error out"=w509:errorcluster)  [unwired: 17 in]
            }
          }
          n149 = call "BaseProcess.set event status.vi"("i ref in"=w475, "EventStatus"=w472, "error in (no error)"=w474) -> ("i ref out"=w471:refnum<vi>, "error out"=w473:errorcluster)  [unwired: 14 in, 1 out]
          n150 = Unbundle By Name(w473) -> ("source"=w464:string, "code"=w479:i32)
          n151 = call-poly "CoreLib.data 2 byte array.vi"("string"=w464) -> ("byteArray out"=w476:T1)  [unwired: 18 in]
          n152 = Bundle By Name(cluster=w478, "Data"=w476, "Error #"=w479, "Data Descriptor"="C:N") -> (w477:T2)
        }
      }
      n153 = case "Default?" shown="False" w11 {
        tunnel: w12 -> [w21 _]
        tunnel: w10 -> [w20 _]
        frame False {
          n154 = call "DeviceBase.set device state.vi"("i ref in"=w20, "implicit"=TRUE, "device error"=w21) -> ()  [unwired: 14 in, 3 out]
        }
        frame True {
        }
      }
    }
    frame Error {
    }
  }
  "answer cluster" <- w3
  "i ref out" <- w1
  "error out" <- w2
